vi "周期设置.vi"(11 "定时控制参数输入":T1) -> (3 "定时控制参数输出":T1)   [LabVIEW 2016, in "质控单元.lvlib"]
uses:
  <vilib>/Utility/miscctls.llb/LVPointTypeDef.ctl
panel:
  in  "采配水启用":bool
  in  "模块选择":T2
  in  "确定":bool
  in  "取消":bool
  in  "定时功能启用":bool
  out "选项卡控件":enum32{"定点启动", "间隔启动"}(tab)
  in  "24H周期设置":bool[](xcontrol)
  in  "已经启动次数":dbl
  in  "设定启动次数":dbl
  in  "定时间隔":dbl
  in  "周期设置类型":enum16{"定点启动", "间隔启动"}(ring)
  # "仪器测试类型："
  # "周期设置类型："
  # "请输入定时启动间隔"
  # "min"
  # "次"
  # "次"
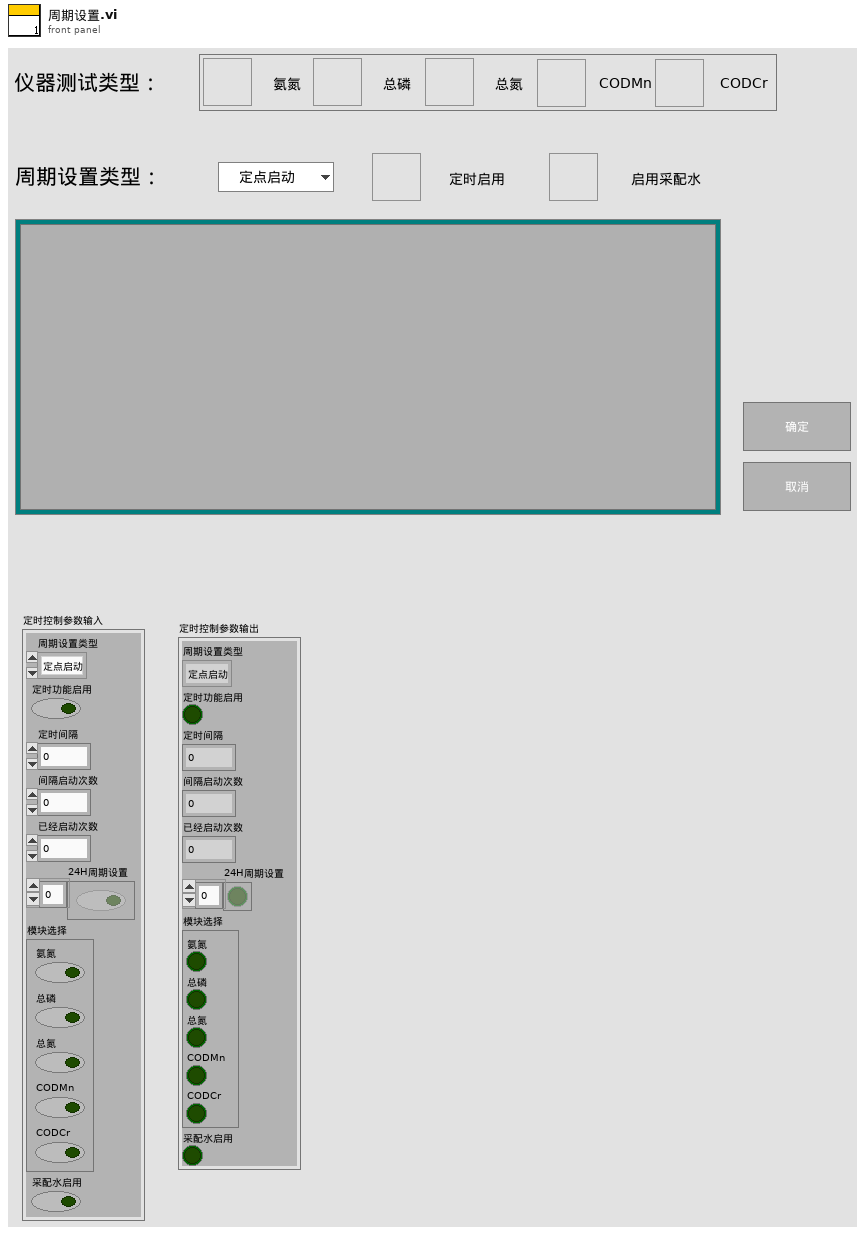
[diagram p1: front panel]
types:
  T1 = cluster{"周期设置类型":enum16{"定点启动", "间隔启动"}, "定时功能启用":bool, "定时间隔":dbl, "间隔启动次数":dbl, "已经启动次数":dbl, "24H周期设置":bool[], "模块选择":cluster{"氨氮":bool, "总磷":bool, "总氮":bool, "CODMn":bool, "CODCr":bool}, "采配水启用":bool}
  T2 = cluster{"氨氮":bool, "总磷":bool, "总氮":bool, "CODMn":bool, "CODCr":bool}
  T3 = typedef "LVPointTypeDef.ctl" = cluster{"Horizontal":i16, "Vertical":i16}
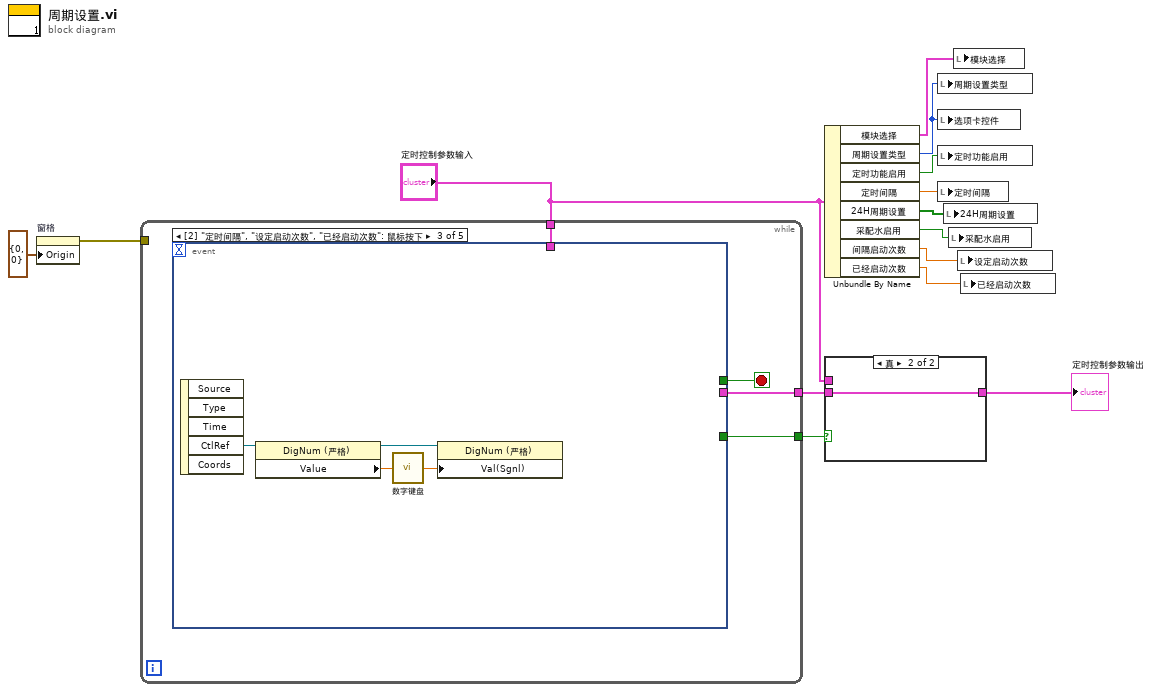
[diagram p0: block diagram]
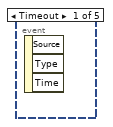
[diagram p3: hidden frame]
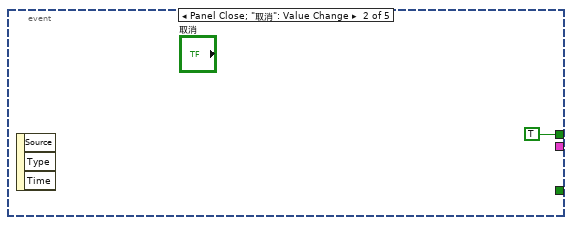
[diagram p4: hidden frame]
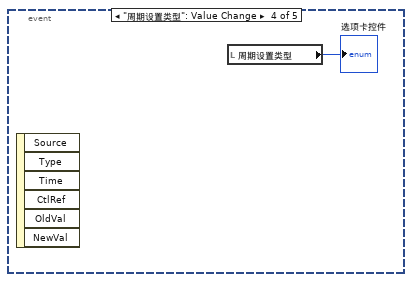
[diagram p5: hidden frame]
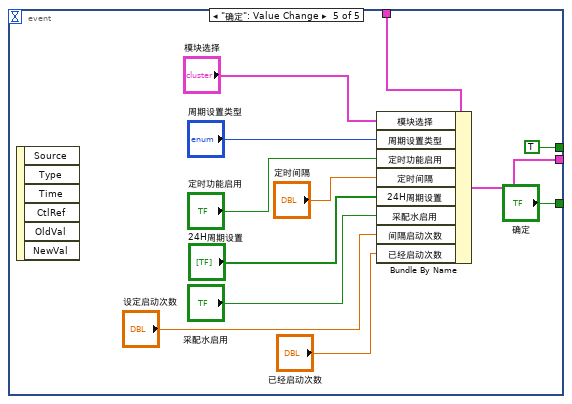
[diagram p6: hidden frame]
diagram:
  n1 = property on="窗格" class="Pane"("Origin"=T3 {"Horizontal"=0, "Vertical"=0} ("原点")) -> (error out=w3:errorcluster)  [unwired: 2 in, 1 out]
  n2 = while {
    tunnel: [w17] -> w9
    tunnel: [w16] -> w10
    tunnel: "定时控制参数输入" -> [w15]
    tunnel: w3 -> [_]
    stop <- w18 stop-if-true
    n3 = event shown="[2] \"定时间隔\", \"设定启动次数\", \"已经启动次数\": 鼠标按下" {
      selector: _ -> [_ _ _ _ _]
      dyn-events: _ -> [_ _ _ _ _]
      timeout: _ -> [_ _ _ _ _]
      tunnel: [_ TRUE _ _ TRUE] -> w18
      tunnel: [_ _ _ _ w32] -> w17
      tunnel: [_ _ _ _ "确定"] -> w16
      tunnel: w15 -> [_ _ _ _ w27]
      event Timeout {
        n4 = event-data() -> ()  [unwired: 1 in, 3 out]
      }
      event Panel Close; "取消": Value Change {
        n5 = event-data() -> ()  [unwired: 1 in, 3 out]
      }
      event "定时间隔", "设定启动次数", "已经启动次数": Mouse Down {
        n6 = event-data() -> ("CtlRef"=w23:refnum<vi>)  [unwired: 1 in, 4 out]
        n7 = property class="DigNum (严格)"(reference=w23) -> (reference out=w20:refnum<vi>, "Value"=w22:dbl)  [unwired: 1 in, 1 out]
        n8 = call "数字键盘.vi"("OldNumber"=w22) -> ("NewNumber"=w21:sgl)
        n9 = property class="DigNum (严格)"(reference=w20, "Val(Sgnl)"=w21) -> ()  [unwired: 1 in, 2 out]
      }
      event "周期设置类型": Value Change {
        n10 = event-data() -> ()  [unwired: 1 in, 6 out]
        n11 = local read "周期设置类型"() -> (→"选项卡控件":enum16{"定点启动", "间隔启动"})
      }
      event "确定": Value Change {
        n12 = event-data() -> ()  [unwired: 1 in, 6 out]
        n13 = Bundle By Name(cluster=w27, "模块选择"="模块选择", "周期设置类型"="周期设置类型", "定时功能启用"="定时功能启用", "定时间隔"="定时间隔", "24H周期设置"="24H周期设置", "采配水启用"="采配水启用", "间隔启动次数"="设定启动次数", "已经启动次数"="已经启动次数") -> (w32:T1)
      }
    }
  }
  n14 = Unbundle By Name("定时控制参数输入") -> ("模块选择"=w8:T2, "周期设置类型"=w11:enum16{"定点启动", "间隔启动"}, "定时功能启用"=w14:bool, "定时间隔"=w13:dbl, "24H周期设置"=w12:bool[], "采配水启用"=w6:bool, "间隔启动次数"=w2:dbl, "已经启动次数"=w1:dbl)
  n15 = case shown="真" w10 {
    tunnel: w9 -> [_ w38]
    tunnel: [w37 w38] -> w7
    tunnel: "定时控制参数输入" -> [w37 _]
    frame False {
    }
    frame True {
    }
  }
  "定时控制参数输出" <- w7
  n16 = local write "周期设置类型"(w11) -> ()
  n17 = local write "选项卡控件"(w11) -> ()
  n18 = local write "定时功能启用"(w14) -> ()
  n19 = local write "定时间隔"(w13) -> ()
  n20 = local write "24H周期设置"(w12) -> ()
  n21 = local write "采配水启用"(w6) -> ()
  n22 = local write "模块选择"(w8) -> ()
  n23 = local write "设定启动次数"(w2) -> ()
  n24 = local write "已经启动次数"(w1) -> ()
